vi "_FPGA Check Source ID.vi"(1 "error in (no error)":errorcluster) -> (0 "Source ID OK":bool)   [LabVIEW 2012]
uses:
  _RT Global.vi
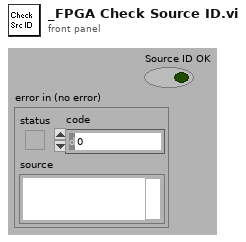
[diagram p1: front panel]
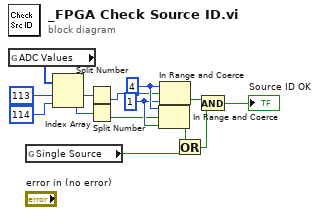
[diagram p0: block diagram]
diagram:
  w14 = u16 4 ("upper limit")
  w13 = u16 1 ("lower limit")
  n1 = global read "_RT Global.vi" "ADC Values"() -> (w4:i32[])
  n2 = global read "_RT Global.vi" "Single Source"() -> (w3:bool)
  n3 = Index Array(array=w4, index #1=113 ("ADC Channel (64)"), index #2=114 ("ADC Channel (64)")) -> (element #1=w7:i32, element #2=w8:i32)
  n4 = Split Number(x=w7) -> (lo(x)=w10:u16)  [unwired: 1 out]
  n5 = Split Number(x=w8) -> (lo(x)=w12:u16)  [unwired: 1 out]
  n6 = In Range and Coerce(upper limit=w14, x=w12, lower limit=w13) -> (In Range?=w2:bool)  [unwired: 1 out]
  n7 = In Range and Coerce(upper limit=w14, x=w10, lower limit=w13) -> (In Range?=w11:bool)  [unwired: 1 out]
  n8 = Or(x=w2, y=w3) -> (x .or. y?=w1:bool)
  n9 = And(x=w11, y=w1) -> (x .and. y?=→"Source ID OK":bool)
